vi "Configure Sequence (Step).vi"(0 "VISA resource name":refnum<visa-resource-name>, 1 "Channel Name (1)":string="1", 4 "Waveform Type (1: Voltage)":i32(ring)=1 items=["Voltage"=1, "Current"=0], 5 "error in (no error)":errorcluster {"code" format="%.0x"}, 6 "Step Sequence  Start Time (0.0 s)":dbl format="%^.3e", 7 "Step Sequence  End Time (0.0 s)":dbl format="%^.3e", 8 "Step Sequence Start Level (0.0)":dbl format="%^.3e", 9 "Step Sequence  End Level (0.0)":dbl format="%^.3e", 12 "Sequence Step Number (0)":i32) -> (14 "VISA resource name out":refnum<visa-resource-name>, 19 "error out":errorcluster {"code" format="%.0x"})   [LabVIEW 2010, in "Agilent N6700 Series.lvlib"]
doc: "This VI configures the step sequence.\n\n<b>Note:</b>\n\nSequence capability is only available on the N6705B DC Power Analyzer."
uses:
  Agilent N6700 Series.lvlib
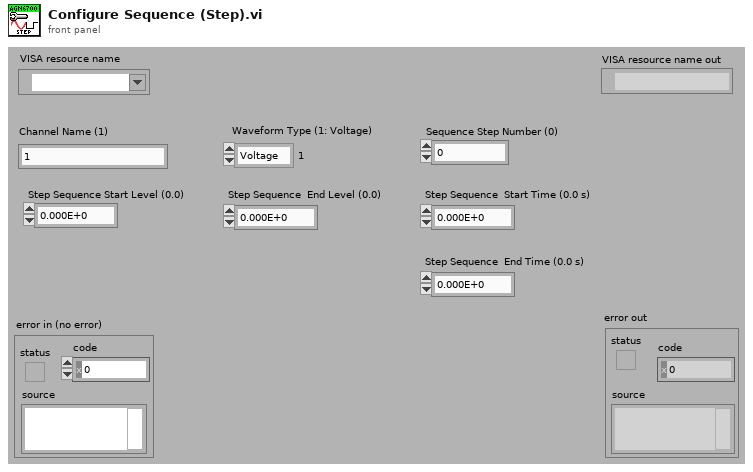
[diagram p1: front panel]
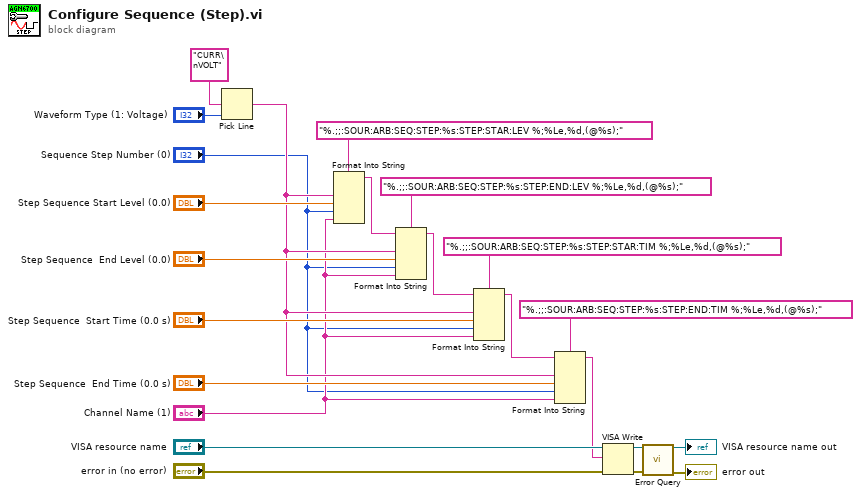
[diagram p0: block diagram]
diagram:
  n1 = Pick Line(multi-line string="CURR\nVOLT", line index="Waveform Type (1: Voltage)") -> (output string=w3:string)  [unwired: 1 in]
  n2 = Format Into String(format string="%.;;:SOUR:ARB:SEQ:STEP:%s:STEP:STAR:LEV %;%Le,%d,(@%s);", w3, "Step Sequence Start Level (0.0)", "Sequence Step Number (0)", "Channel Name (1)") -> (resulting string=w13:string)  [unwired: 2 in, 1 out]
  n3 = Format Into String(format string="%.;;:SOUR:ARB:SEQ:STEP:%s:STEP:END:LEV %;%Le,%d,(@%s);", initial string=w13, w3, "Step Sequence  End Level (0.0)", "Sequence Step Number (0)", "Channel Name (1)") -> (resulting string=w12:string)  [unwired: 1 in, 1 out]
  n4 = Format Into String(format string="%.;;:SOUR:ARB:SEQ:STEP:%s:STEP:STAR:TIM %;%Le,%d,(@%s);", initial string=w12, w3, "Step Sequence  Start Time (0.0 s)", "Sequence Step Number (0)", "Channel Name (1)") -> (resulting string=w5:string)  [unwired: 1 in, 1 out]
  n5 = Format Into String(format string="%.;;:SOUR:ARB:SEQ:STEP:%s:STEP:END:TIM %;%Le,%d,(@%s);", initial string=w5, w3, "Step Sequence  End Time (0.0 s)", "Sequence Step Number (0)", "Channel Name (1)") -> (resulting string=w4:string)  [unwired: 1 in, 1 out]
  n6 = VISA Write(VISA resource name="VISA resource name", write buffer=w4, error in (no error)="error in (no error)") -> (VISA resource name out=w19:refnum<visa-resource-name>, error out=w18:errorcluster)  [unwired: 1 out]
  n7 = call "Error Query.vi"("VISA resource name"=w19, "error in (no error)"=w18) -> ("VISA resource name out"=→"VISA resource name out":refnum<visa-resource-name>, "error out"=→"error out":errorcluster)  [unwired: 10 in, 2 out]
